vi "PB_add_VLIW.vi"(4 "Use Global (F)?":bool, 5 "Definitions":T1={"External MemorySize"=32768, "Internal Memory Size"=512, "Overhead Ticks"=3, "Min Delay Loops"=3, "Loop Count Correction"=1, "Long Delay Loop Count Correction"=2, "Min Instruction Ticks"=6, "Long Delay Ticks"=4294967295, "Clock Period (s)"=1e-08, "Overhead Time (s)"=3e-08, "Min Instruction Cycle Time (s)"=9e-08, "Long Delay Time (s) "=42.94967298} {"Long Delay Time (s)" format="%.8p"; "Min Instruction Cycle Time (s)" format="%.0p"; "Overhead Time (s)" format="%.0p"; "Clock Period (s)" format="%.0p"; "Long Delay Ticks" format="%.0x"}, 6 "OP code":u8(ring) items=["Continue", "Stop", "Loop", "End Loop", "Jump", "Return", "Go To", "Long Delay", "Wait"], 7 "Data Field":u32, 8 "error in (no error)":errorcluster, 9 "Delay":dbl=50.0 format="%.3p", 10 "Digital Bits":u32 format="%.0x", 11 "VLIW Array In":T2(array[cluster]) {"OP Code" format="%.0x"; "Output Bits" format="%.0x"}) -> (0 "error out":errorcluster, 1 "Actual Delay":dbl=50.0 format="%.2p", 3 "VLIW Array Out":T2(array[cluster])=[{"Output Bits"=0, "Data Field"=3, "OP Code"=2, "Delay Count"=4}, {"Output Bits"=0, "Data Field"=0, "OP Code"=3, "Delay Count"=4}, {"Output Bits"=0, "Data Field"=0, "OP Code"=0, "Delay Count"=2599999997}, {"Output Bits"=0, "Data Field"=2, "OP Code"=7, "Delay Count"=1073741821}, {"Output Bits"=0, "Data Field"=0, "OP Code"=0, "Delay Count"=705032701}] {"OP Code" format="%.0x"; "Output Bits" format="%.0x"})   [LabVIEW 2013, in "PulseBlaster.lvlib"]
doc: "This vi writes a single command to \"VLIW Array\", where \"VLIW array\" is an array of clusters which contain an image of the command array of the PulseBlaster.\n\nIt provides some error checking on the inputs to help make sure you won't confuse the PulseBlaster.\nInputs:\n 1) Digital Bits (24 bit output flags)\n 2) Data Field (24 bits)\n 3) OP Code (4 bits)\n 4) Delay (in units of seconds)\n 5) error in.\n 6) Input array (The array to be appended to.)\nOutputs\n 1) Actual Delay (in units of seconds, rounded to nearest 10ns)\n 2) error out.\n 3) Output array. (The appended array.)\n\n\"PB_add_VLIW\" uses the globally defined variables in \"PB_defines\". The long delay command should be entirely transparent, so the user does not need to envoke it.\n\nFor New SetList, PB_defines have been superceeded by object data and are passed in as \"definitions.\""
uses:
  PulseBlaster.lvlib
  PB_defines.vi
panel:
  # "append"
  # "to"
  # "PB_add_VLIW has been using global definitions.\nHowever, we'd like it to use PulseBlaster\nprivate data as these are now part of the object.\n\nFor now, leave use Global as option for manual controls..."
  # "(Period*Long D Ticks)+Overhead time"
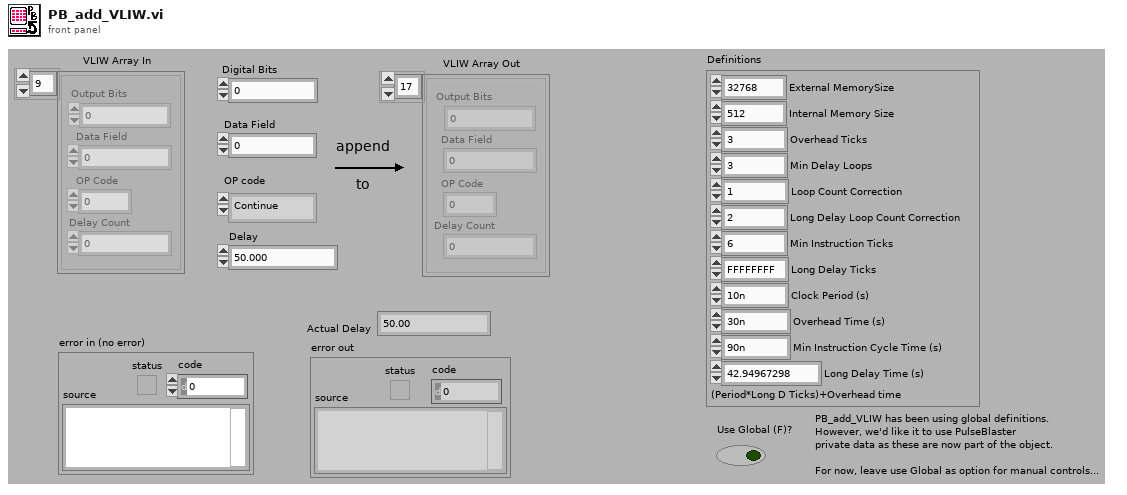
[diagram p1: front panel]
types:
  T1 = cluster{"External MemorySize":u16, "Internal Memory Size":u16, "Overhead Ticks":u8, "Min Delay Loops":u8, "Loop Count Correction":u8, "Long Delay Loop Count Correction":u8, "Min Instruction Ticks":u8, "Long Delay Ticks":u64, "Clock Period (s)":dbl, "Overhead Time (s)":dbl, "Min Instruction Cycle Time (s)":dbl, "Long Delay Time (s) ":dbl}
  T2 = cluster{"Output Bits":u32, "Data Field":u32, "OP Code":u8, "Delay Count":u64}[]
  T3 = cluster{"Output Bits":u32, "Data Field":u32, "OP Code":u8, "Delay Count":u64}
  T4 = cluster{"Digital Bits":u32, "Data Field":u32, "OP code":u8, u64}
  T5 = cluster{"Digital Bits":u32, "Data Field":u32, "OP code":u8, "Delay Count":u64}[]
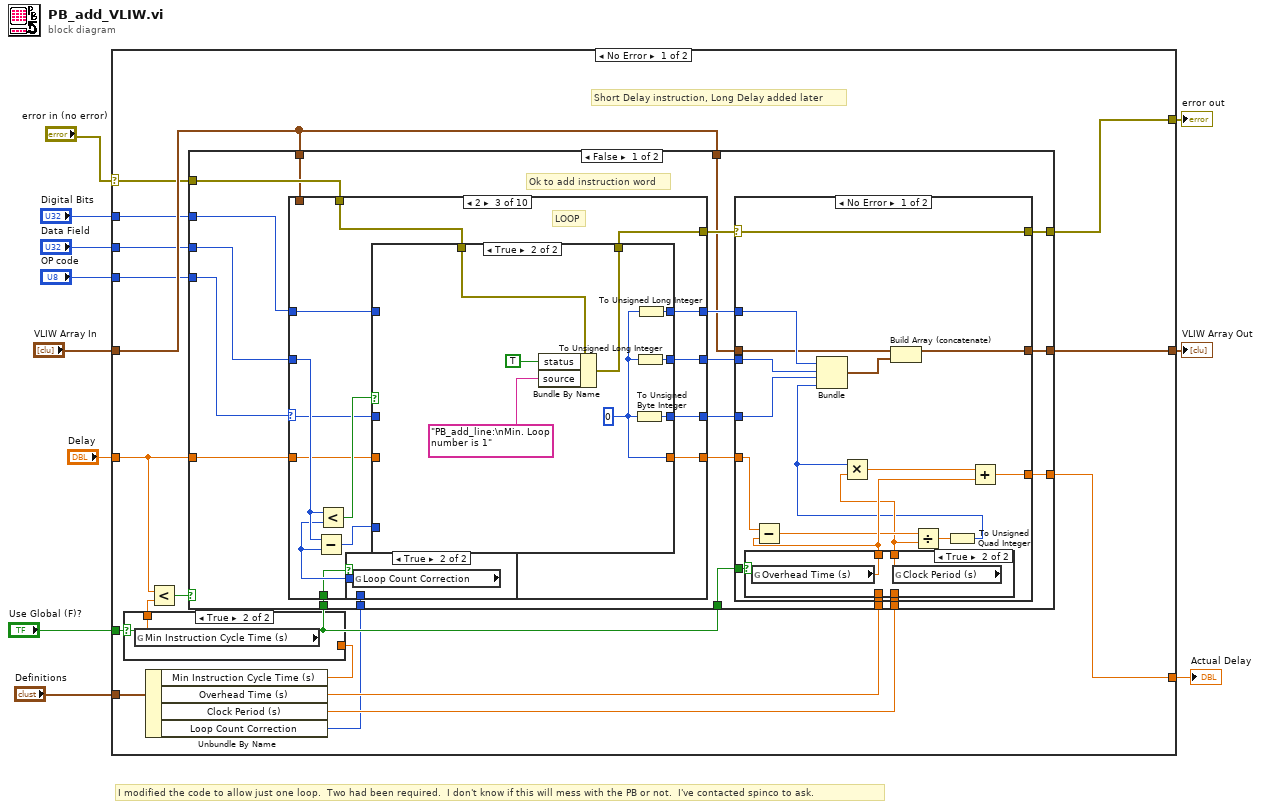
[diagram p0: block diagram]
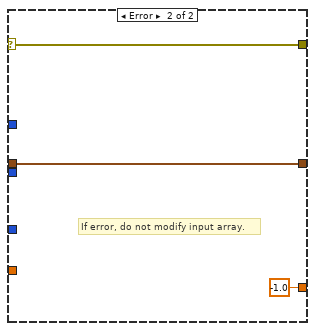
[diagram p4: hidden frame]
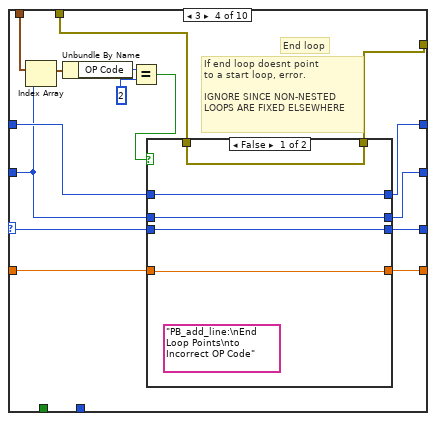
[diagram p9: hidden frame]
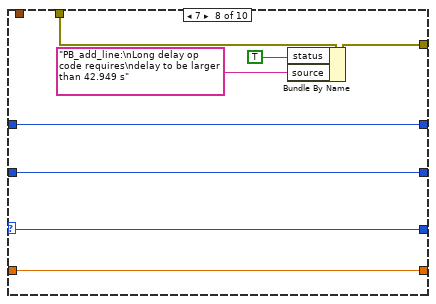
[diagram p14: hidden frame]
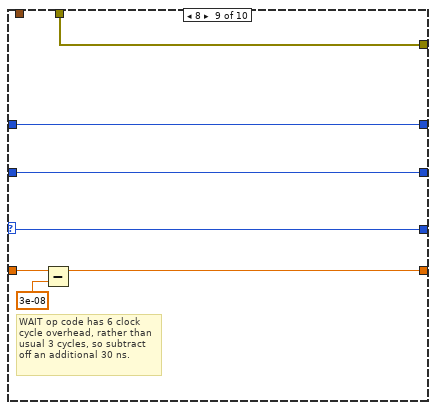
[diagram p15: hidden frame]
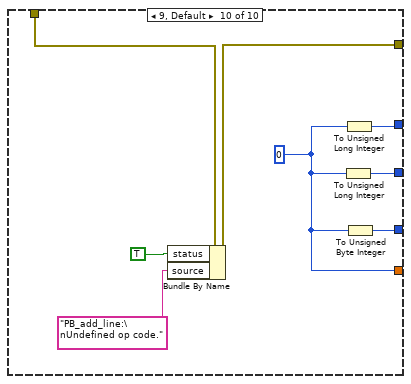
[diagram p16: hidden frame]
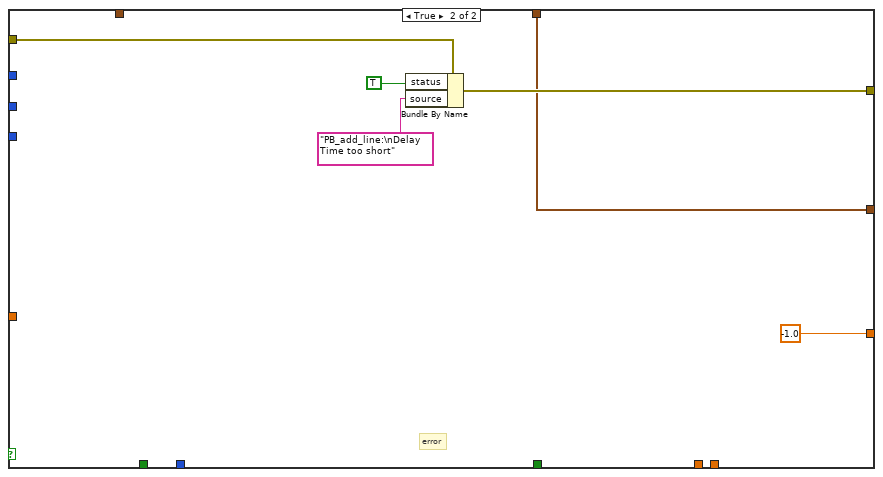
[diagram p17: hidden frame]
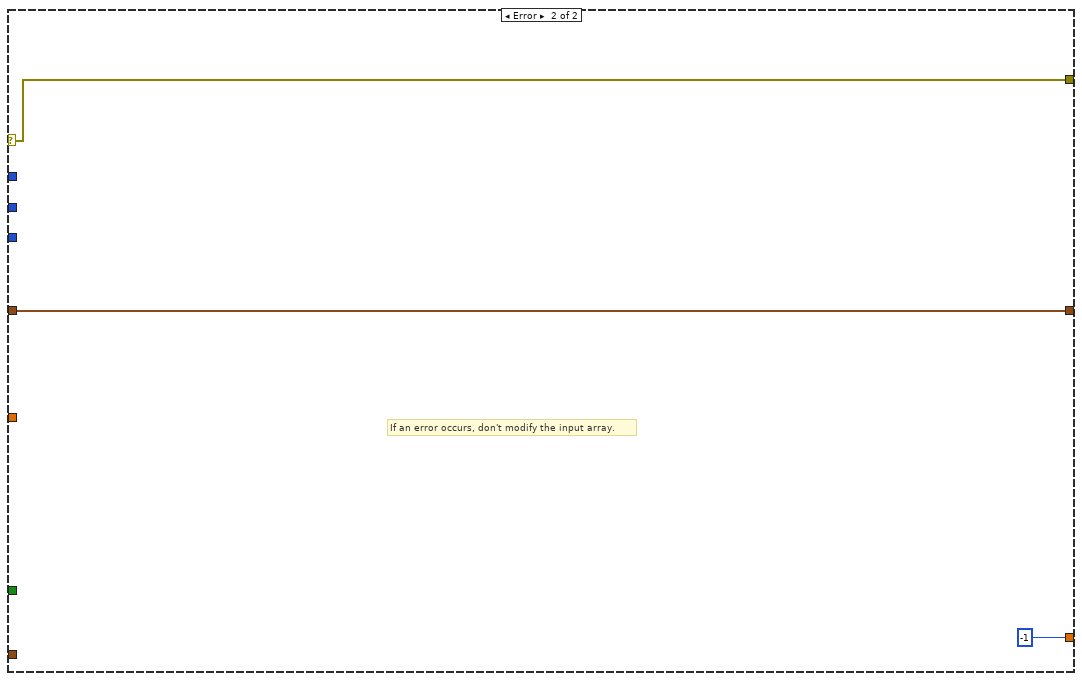
[diagram p18: hidden frame]
diagram:
  # "I modified the code to allow just one loop.  Two had been required.  I don't know if this will mess with the PB or not.  I've contacted spinco to ask."
  n1 = case shown="No Error" "error in (no error)" {
    selector: "error in (no error)" -> [w18 w185]
    tunnel: [w28 w185] -> w11
    tunnel: [w27 -1] -> w9
    tunnel: [w26 w186] -> w8
    tunnel: "VLIW Array In" -> [w25 w186]
    tunnel: "Digital Bits" -> [w24 _]
    tunnel: "Data Field" -> [w23 _]
    tunnel: "OP code" -> [w22 _]
    tunnel: "Delay" -> [w19 _]
    tunnel: "Definitions" -> [w17 _]
    tunnel: "Use Global (F)?" -> [w13 _]
    frame No Error {
      # "Short Delay instruction, Long Delay added later"
      n2 = Unbundle By Name(w17) -> ("Min Instruction Cycle Time (s)"=w16:dbl, "Overhead Time (s)"=w15:dbl, "Clock Period (s)"=w14:dbl, "Loop Count Correction"=w12:u8)
      n3 = case shown="True" w13 {
        tunnel: [w29 w30] -> w21
        tunnel: w16 -> [w29 _]
        frame False {
        }
        frame True {
          n4 = global read "PB_defines.vi" "Min Instruction Cycle Time (s)"() -> (w30:dbl)
        }
      }
      n5 = Less?(x=w19, y=w21) -> (x < y?=w20:bool)
      n6 = case shown="False" w20 {
        tunnel: w18 -> [w50 w184]
        tunnel: [w49 w183] -> w28
        tunnel: [w43 -1.0] -> w27
        tunnel: w19 -> [w42 _]
        tunnel: [w41 w180] -> w26
        tunnel: w25 -> [w40 w180]
        tunnel: w24 -> [w39 _]
        tunnel: w23 -> [w38 _]
        tunnel: w22 -> [w37 _]
        tunnel: w25 -> [w36 _]
        tunnel: w13 -> [w35 _]
        tunnel: w15 -> [w34 _]
        tunnel: w14 -> [w33 _]
        tunnel: w13 -> [w32 _]
        tunnel: w12 -> [w31 _]
        frame False {
          # "Ok to add instruction word"
          n7 = case shown="2" w37 {
            selector: w37 -> [w76 w81 w88 w116 w141 w146 w151 w156 w164 _]
            tunnel: w50 -> [w80 w82 w97 w127 w145 w147 w152 w162 w170 w175]
            tunnel: [w80 w82 w96 w128 w145 w147 w152 w161 w170 w176] -> w44
            tunnel: [w79 w85 w95 w123 w144 w150 w155 w160 w169 w172] -> w48
            tunnel: w39 -> [w79 w85 w91 w126 w144 w150 w155 w160 w169 _]
            tunnel: [w78 w84 w94 w122 w143 w149 w154 w159 w168 w171] -> w47
            tunnel: w38 -> [w78 w84 w100 w125 w143 w149 w154 w159 w168 _]
            tunnel: [w76 w81 w93 w121 w141 w146 w151 w156 w164 w173] -> w46
            tunnel: [w77 w83 w92 w120 w142 w148 w153 w158 w165 w174] -> w45
            tunnel: w42 -> [w77 w83 w90 w124 w142 w148 w153 w158 w166 _]
            tunnel: w36 -> [_ _ _ w117 _ _ _ _ _ _]
            tunnel: w32 -> [_ _ w87 _ _ _ _ _ _ _]
            tunnel: w31 -> [_ _ w86 _ _ _ _ _ _ _]
            frame 0 {
              # "Continue"
            }
            frame 1 {
              # "Stop"
            }
            frame 2 {
              # "LOOP"
              n8 = case shown="True" w87 {
                tunnel: [w101 w102] -> w99
                tunnel: w86 -> [w101 _]
                frame False {
                }
                frame True {
                  n9 = global read "PB_defines.vi" "Loop Count Correction"() -> (w102:u8)
                }
              }
              n10 = Subtract(x=w100, y=w99) -> (x-y=w89:u32)
              n11 = Less?(x=w100, y=w99) -> (x < y?=w98:bool)
              n12 = case shown="True" w98 {
                tunnel: w97 -> [w107 w113]
                tunnel: [w107 w112] -> w96
                tunnel: [w106 w108] -> w95
                tunnel: [w105 w109] -> w94
                tunnel: [w103 w110] -> w93
                tunnel: [w104 w111] -> w92
                tunnel: w91 -> [w106 _]
                tunnel: w89 -> [w105 _]
                tunnel: w90 -> [w104 _]
                tunnel: w88 -> [w103 _]
                frame False {
                }
                frame True {
                  w111 = 0
                  n13 = Bundle By Name(cluster=w113, "status"=TRUE, "source"="PB_add_line:\nMin. Loop number is 1") -> (w112:errorcluster)
                  n14 = To Unsigned Byte Integer(number=w111) -> (unsigned 8bit integer=w110:u8)
                  n15 = To Unsigned Long Integer(number=w111) -> (unsigned 32bit integer=w109:u32)
                  n16 = To Unsigned Long Integer(number=w111) -> (unsigned 32bit integer=w108:u32)
                }
              }
            }
            frame 3 {
              # "If end loop doesnt point\nto a start loop, error.\n\nIGNORE SINCE NON-NESTED\nLOOPS ARE FIXED ELSEWHERE"
              # "End loop"
              n17 = Index Array(array=w117, index=w125) -> (element=w119:T3)
              n18 = Unbundle By Name(w119) -> ("OP Code"=w118:u8)
              n19 = Equal?(x=w118, y=2) -> (x = y?=w129:bool)
              n20 = case shown="False" w129 {
                tunnel: [w131 w140] -> w128
                tunnel: w127 -> [w131 w140]
                tunnel: w126 -> [w133 w138]
                tunnel: w125 -> [w135 w137]
                tunnel: [w135 w137] -> w122
                tunnel: w116 -> [w132 w136]
                tunnel: w124 -> [w134 w139]
                tunnel: [w134 w139] -> w120
                tunnel: [w133 w138] -> w123
                tunnel: [w132 w136] -> w121
                frame False {
                  (unwired) "PB_add_line:\nEnd Loop Points\nto Incorrect OP Code"
                }
                frame True {
                }
              }
            }
            frame 4 {
            }
            frame 5 {
            }
            frame 6 {
            }
            frame 7 {
              n21 = Bundle By Name(cluster=w162, "status"=TRUE, "source"="PB_add_line:\nLong delay op code requires\ndelay to be larger than 42.949 s") -> (w161:errorcluster)
            }
            frame 8 {
              # "WAIT op code has 6 clock\ncycle overhead, rather than\nusual 3 cycles, so subtract\noff an additional 30 ns."
              n22 = Subtract(x=w166, y=3e-08) -> (x-y=w165:dbl)
            }
            frame 9, Default {
              w174 = 0
              n23 = Bundle By Name(cluster=w175, "status"=TRUE, "source"="PB_add_line:\nUndefined op code.") -> (w176:errorcluster)
              n24 = To Unsigned Long Integer(number=w174) -> (unsigned 32bit integer=w171:u32)
              n25 = To Unsigned Long Integer(number=w174) -> (unsigned 32bit integer=w172:u32)
              n26 = To Unsigned Byte Integer(number=w174) -> (unsigned 8bit integer=w173:u8)
            }
          }
          n27 = case shown="No Error" w44 {
            selector: w44 -> [w54 w73]
            tunnel: [w54 w73] -> w49
            tunnel: w48 -> [w61 _]
            tunnel: w47 -> [w62 _]
            tunnel: w46 -> [w63 _]
            tunnel: w45 -> [w64 _]
            tunnel: [w57 -1.0] -> w43
            tunnel: [w56 w74] -> w41
            tunnel: w40 -> [w55 w74]
            tunnel: w35 -> [w53 _]
            tunnel: w34 -> [w52 _]
            tunnel: w33 -> [w51 _]
            frame No Error {
              n28 = case shown="True" w53 {
                tunnel: [w70 w72] -> w68
                tunnel: [w69 w71] -> w66
                tunnel: w52 -> [w70 _]
                tunnel: w51 -> [w69 _]
                frame False {
                }
                frame True {
                  n29 = global read "PB_defines.vi" "Overhead Time (s)"() -> (w72:dbl)
                  n30 = global read "PB_defines.vi" "Clock Period (s)"() -> (w71:dbl)
                }
              }
              n31 = Subtract(x=w64, y=w68) -> (x-y=w67:dbl)
              n32 = Divide(x=w67, y=w66) -> (x/y=w65:dbl)
              n33 = To Unsigned Quad Integer(1:w65) -> (0:w59:u64)
              n34 = Bundle("Digital Bits"=w61, "Data Field"=w62, "OP code"=w63, w59) -> (w60:T4)  [unwired: 1 out]
              n35 = Multiply(x=w59, y=w66) -> (x*y=w58:dbl)
              n36 = Build Array (concatenate)(w55, w60) -> (w56:T5)
              n37 = Add(x=w58, y=w68) -> (x+y=w57:dbl)
            }
            frame Error {
              # "If error, do not modify input array."
            }
          }
        }
        frame True {
          # "error"
          n38 = Bundle By Name(cluster=w184, "status"=TRUE, "source"="PB_add_line:\nDelay Time too short") -> (w183:errorcluster)
        }
      }
    }
    frame Error {
      # "If an error occurs, don't modify the input array."
    }
  }
  "error out" <- w11
  "Actual Delay" <- w9
  "VLIW Array Out" <- w8
